vi "Waveform 8 channels LP pt by pt 1.vi"(6 "order":i32=2, 8 "fl":dbl, 10 "fs":dbl, 11 "Array in":waveform(dbl)[](array[waveform])) -> (3 "Array out":waveform(dbl)[](array[waveform]))   [LabVIEW 2013]
uses:
  <vilib>/Analysis/3filter.llb/Filter Passband Type.ctl
  <vilib>/ptbypt/NI_PtbyPt.lvlib
  <vilib>/Analysis/NI_AALBase.lvlib
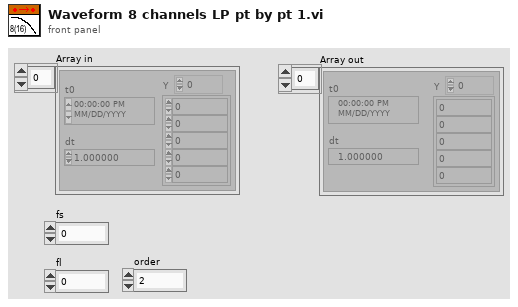
[diagram p1: front panel]
types:
  T1 = typedef "NI_AALBase.lvlib/Filter Passband Type.ctl" = enum32{"Lowpass", "Highpass", "Bandpass", "Bandstop"}
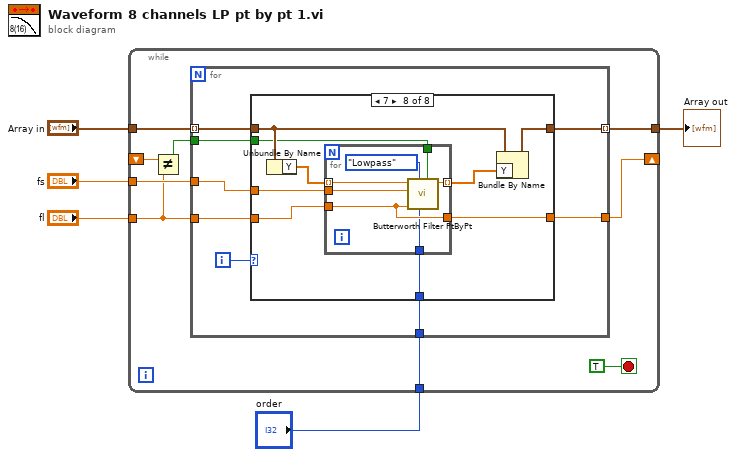
[diagram p0: block diagram]
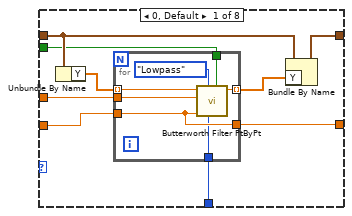
[diagram p2: hidden frame]
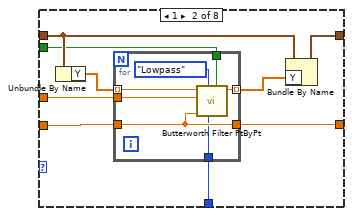
[diagram p3: hidden frame]
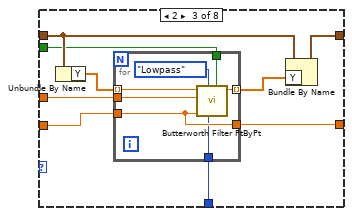
[diagram p4: hidden frame]
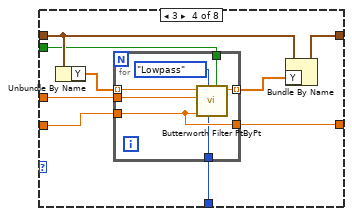
[diagram p5: hidden frame]
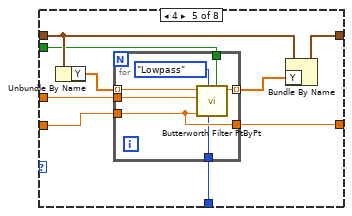
[diagram p6: hidden frame]
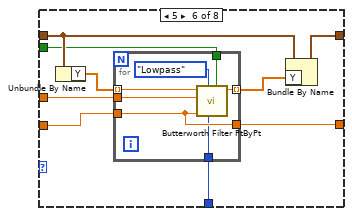
[diagram p7: hidden frame]
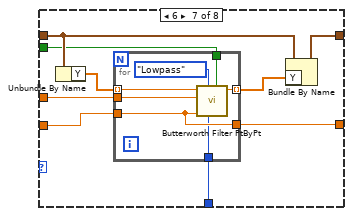
[diagram p8: hidden frame]
diagram:
  n1 = while {
    tunnel: "Array in" -> [w14]
    tunnel: [w13] -> w4
    tunnel: "fs" -> [w10]
    tunnel: "fl" -> [w7]
    shift-right: [w11] -> _
    shift-left: _ -> [w9]
    tunnel: "order" -> [w8]
    stop <- TRUE stop-if-true
    n2 = Not Equal?(x=w9, y=w7) -> (x != y?=w6:bool)
    n3 = for {
      tunnel: w14 -> [w20] mode=indexing
      tunnel: w10 -> [w22]
      tunnel: [w21] -> w13 mode=indexing
      tunnel: w7 -> [w19]
      tunnel: [w17] -> w11
      tunnel: w6 -> [w16]
      tunnel: w8 -> [w15]
      i -> [w18]
      n4 = case shown="7" w18 {
        tunnel: w22 -> [w27 w43 w59 w75 w91 w107 w123 w139]
        tunnel: [w31 w47 w63 w79 w95 w111 w127 w143] -> w21
        tunnel: w20 -> [w29 w45 w61 w77 w93 w109 w125 w141]
        tunnel: [w30 w46 w62 w78 w94 w110 w126 w142] -> w17
        tunnel: w19 -> [w26 w42 w58 w74 w90 w106 w122 w138]
        tunnel: w16 -> [w24 w40 w56 w72 w88 w104 w120 w136]
        tunnel: w15 -> [w23 w39 w55 w71 w87 w103 w119 w135]
        frame 0, Default {
          n5 = Unbundle By Name(w29) -> ("Y"=w25:dbl[])
          n6 = for {
            tunnel: w25 -> [w38] mode=indexing
            tunnel: w26 -> [w35]
            tunnel: w27 -> [w37]
            tunnel: [w36] -> w28 mode=indexing
            tunnel: [w35] -> w30
            tunnel: w24 -> [w33]
            tunnel: w23 -> [w32]
            n7 = call <vilib>:"Butterworth Filter PtByPt.vi"("initialize"=w33, "order"=w32, "filter type"=Filter_Passband_Type."Lowpass", "low cutoff freq: fl"=w35, "sampling freq: fs"=w37, "x"=w38) -> ("Filtered x"=w36:dbl)  [unwired: 3 in, 1 out]
          }
          n8 = Bundle By Name(cluster=w29, "Y"=w28) -> (w31:waveform(dbl))
        }
        frame 1 {
          n9 = Unbundle By Name(w45) -> ("Y"=w41:dbl[])
          n10 = for {
            tunnel: w41 -> [w54] mode=indexing
            tunnel: w42 -> [w51]
            tunnel: w43 -> [w53]
            tunnel: [w52] -> w44 mode=indexing
            tunnel: [w51] -> w46
            tunnel: w40 -> [w49]
            tunnel: w39 -> [w48]
            n11 = call <vilib>:"Butterworth Filter PtByPt.vi"("initialize"=w49, "order"=w48, "filter type"=Filter_Passband_Type."Lowpass", "low cutoff freq: fl"=w51, "sampling freq: fs"=w53, "x"=w54) -> ("Filtered x"=w52:dbl)  [unwired: 3 in, 1 out]
          }
          n12 = Bundle By Name(cluster=w45, "Y"=w44) -> (w47:waveform(dbl))
        }
        frame 2 {
          n13 = Unbundle By Name(w61) -> ("Y"=w57:dbl[])
          n14 = for {
            tunnel: w57 -> [w70] mode=indexing
            tunnel: w58 -> [w67]
            tunnel: w59 -> [w69]
            tunnel: [w68] -> w60 mode=indexing
            tunnel: [w67] -> w62
            tunnel: w56 -> [w65]
            tunnel: w55 -> [w64]
            n15 = call <vilib>:"Butterworth Filter PtByPt.vi"("initialize"=w65, "order"=w64, "filter type"=Filter_Passband_Type."Lowpass", "low cutoff freq: fl"=w67, "sampling freq: fs"=w69, "x"=w70) -> ("Filtered x"=w68:dbl)  [unwired: 3 in, 1 out]
          }
          n16 = Bundle By Name(cluster=w61, "Y"=w60) -> (w63:waveform(dbl))
        }
        frame 3 {
          n17 = Unbundle By Name(w77) -> ("Y"=w73:dbl[])
          n18 = for {
            tunnel: w73 -> [w86] mode=indexing
            tunnel: w74 -> [w83]
            tunnel: w75 -> [w85]
            tunnel: [w84] -> w76 mode=indexing
            tunnel: [w83] -> w78
            tunnel: w72 -> [w81]
            tunnel: w71 -> [w80]
            n19 = call <vilib>:"Butterworth Filter PtByPt.vi"("initialize"=w81, "order"=w80, "filter type"=Filter_Passband_Type."Lowpass", "low cutoff freq: fl"=w83, "sampling freq: fs"=w85, "x"=w86) -> ("Filtered x"=w84:dbl)  [unwired: 3 in, 1 out]
          }
          n20 = Bundle By Name(cluster=w77, "Y"=w76) -> (w79:waveform(dbl))
        }
        frame 4 {
          n21 = Unbundle By Name(w93) -> ("Y"=w89:dbl[])
          n22 = for {
            tunnel: w89 -> [w102] mode=indexing
            tunnel: w90 -> [w99]
            tunnel: w91 -> [w101]
            tunnel: [w100] -> w92 mode=indexing
            tunnel: [w99] -> w94
            tunnel: w88 -> [w97]
            tunnel: w87 -> [w96]
            n23 = call <vilib>:"Butterworth Filter PtByPt.vi"("initialize"=w97, "order"=w96, "filter type"=Filter_Passband_Type."Lowpass", "low cutoff freq: fl"=w99, "sampling freq: fs"=w101, "x"=w102) -> ("Filtered x"=w100:dbl)  [unwired: 3 in, 1 out]
          }
          n24 = Bundle By Name(cluster=w93, "Y"=w92) -> (w95:waveform(dbl))
        }
        frame 5 {
          n25 = Unbundle By Name(w109) -> ("Y"=w105:dbl[])
          n26 = for {
            tunnel: w105 -> [w118] mode=indexing
            tunnel: w106 -> [w115]
            tunnel: w107 -> [w117]
            tunnel: [w116] -> w108 mode=indexing
            tunnel: [w115] -> w110
            tunnel: w104 -> [w113]
            tunnel: w103 -> [w112]
            n27 = call <vilib>:"Butterworth Filter PtByPt.vi"("initialize"=w113, "order"=w112, "filter type"=Filter_Passband_Type."Lowpass", "low cutoff freq: fl"=w115, "sampling freq: fs"=w117, "x"=w118) -> ("Filtered x"=w116:dbl)  [unwired: 3 in, 1 out]
          }
          n28 = Bundle By Name(cluster=w109, "Y"=w108) -> (w111:waveform(dbl))
        }
        frame 6 {
          n29 = Unbundle By Name(w125) -> ("Y"=w121:dbl[])
          n30 = for {
            tunnel: w121 -> [w134] mode=indexing
            tunnel: w122 -> [w131]
            tunnel: w123 -> [w133]
            tunnel: [w132] -> w124 mode=indexing
            tunnel: [w131] -> w126
            tunnel: w120 -> [w129]
            tunnel: w119 -> [w128]
            n31 = call <vilib>:"Butterworth Filter PtByPt.vi"("initialize"=w129, "order"=w128, "filter type"=Filter_Passband_Type."Lowpass", "low cutoff freq: fl"=w131, "sampling freq: fs"=w133, "x"=w134) -> ("Filtered x"=w132:dbl)  [unwired: 3 in, 1 out]
          }
          n32 = Bundle By Name(cluster=w125, "Y"=w124) -> (w127:waveform(dbl))
        }
        frame 7 {
          n33 = Unbundle By Name(w141) -> ("Y"=w137:dbl[])
          n34 = for {
            tunnel: w137 -> [w150] mode=indexing
            tunnel: w138 -> [w147]
            tunnel: w139 -> [w149]
            tunnel: [w148] -> w140 mode=indexing
            tunnel: [w147] -> w142
            tunnel: w136 -> [w145]
            tunnel: w135 -> [w144]
            n35 = call <vilib>:"Butterworth Filter PtByPt.vi"("initialize"=w145, "order"=w144, "filter type"=Filter_Passband_Type."Lowpass", "low cutoff freq: fl"=w147, "sampling freq: fs"=w149, "x"=w150) -> ("Filtered x"=w148:dbl)  [unwired: 3 in, 1 out]
          }
          n36 = Bundle By Name(cluster=w141, "Y"=w140) -> (w143:waveform(dbl))
        }
      }
    }
  }
  "Array out" <- w4
